vi "Wait for motor init.vi"(8 "error in (no error)":errorcluster, 11 "VISA Refnum in":refnum<visa-resource-name>) -> (0 "error out":errorcluster, 2 "Motors ready?":bool, 3 "VISA Refnum out":refnum<visa-resource-name>)   [LabVIEW 2020, in "Arduino-Adafruit stepper.lvlib"]
uses:
  Arduino-Adafruit stepper.lvlib
  1655e6bd-b7e5-4ae9-882c-61f458fcb923.vi
  fde5e98c-c600-49ca-8b42-3760f3fbc248.vi
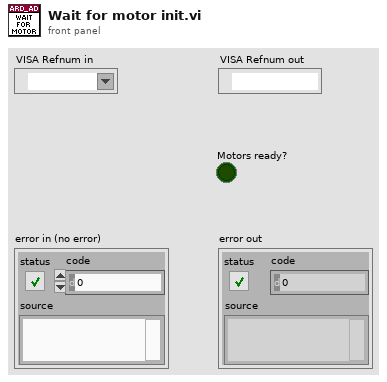
[diagram p1: front panel]
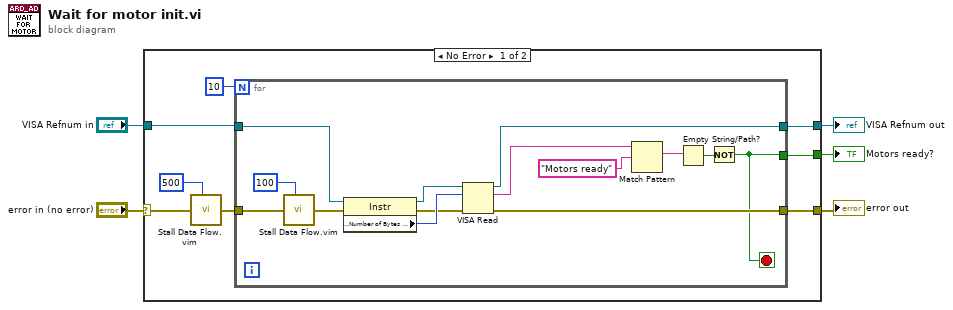
[diagram p0: block diagram]
diagram:
  n1 = case shown="No Error" "error in (no error)" {
    selector: "error in (no error)" -> [w12 w28]
    tunnel: "VISA Refnum in" -> [w13 w29]
    tunnel: [w8 w28] -> w3
    tunnel: [w9 _] -> w2
    tunnel: [w10 w29] -> w1
    frame No Error {
      n2 = call "Stall Data Flow.vim"("value in"=w12, "milliseconds to wait"=u32 500) -> ("value out"=w7:errorcluster)  [unwired: 1 out]
      n3 = for {
        N: 10 -> [_]
        tunnel: [w27] -> w8
        tunnel: w13 -> [w18]
        tunnel: w7 -> [w16]
        tunnel: [w19] -> w9
        tunnel: [w14] -> w10
        stop <- w19 stop-if-true
        n4 = call "Stall Data Flow.vim"("value in"=w16, "milliseconds to wait"=u32 100) -> ("value out"=w15:errorcluster)  [unwired: 1 out]
        n5 = property class="Instr"(reference=w18, error in=w15) -> (reference out=w24:refnum<visa-resource-name>, error out=w25:errorcluster, "Serial Settings:Number of Bytes at Serial Port"=w26:u32)
        n6 = VISA Read(VISA resource name=w24, byte count=w26, error in (no error)=w25) -> (VISA resource name out=w14:refnum<visa-resource-name>, read buffer=w23:string, error out=w27:errorcluster)  [unwired: 1 out]
        n7 = Match Pattern(string=w23, regular expression="Motors ready") -> (match substring=w21:string)  [unwired: 1 in, 3 out]
        n8 = Empty String/Path?(string/path=w21) -> (empty?=w20:bool)
        n9 = Not(x=w20) -> (.not. x?=w19:bool)
      }
    }
    frame Error {
    }
  }
  "error out" <- w3
  "Motors ready?" <- w2
  "VISA Refnum out" <- w1
